vi "Draw.vi"(8 "error in (no error)":errorcluster, 11 "Rectangle in":refnum<class "Rectangle.lvclass">) -> (0 "error out":errorcluster, 2 "Picture":picture, 3 "Rectangle out":refnum<class "Rectangle.lvclass">)   [LabVIEW 2015, in "LV Image Editor Framework.lvlib" / "Rectangle.lvclass"]
uses:
  Rectangle.lvclass
  Shape/Shape.lvclass/Shape.ctl
  Rectangle.lvclass/Rectangle.ctl
  Layered Shape/Layered Shape.lvclass
  Shape/Shape.lvclass
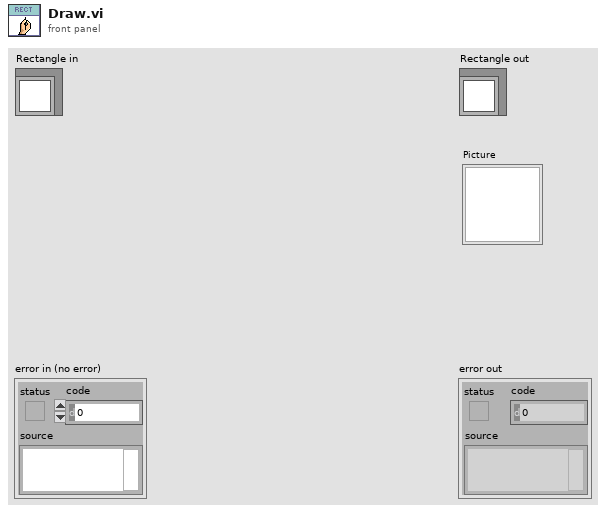
[diagram p1: front panel]
types:
  T1 = cluster{"Left":i32, "Top":i32, "Right":i32, "Bottom":i32}
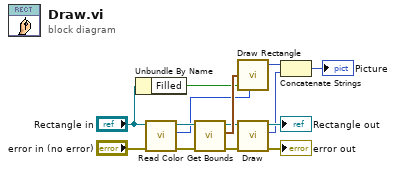
[diagram p0: block diagram]
diagram:
  n1 = Unbundle By Name("Rectangle in") -> ("Filled"=w11:bool)
  n2 = call "Read Color.vi"("error in (no error)"="error in (no error)", "Shape in"="Rectangle in") -> ("error out"=w10:errorcluster, "Color"=w12:u32, "Shape out"=w14:refnum<class "Rectangle.lvclass">)  [unwired: 7 in]
  n3 = call "Get Bounds.vi"("error in (no error)"=w10, "Shape in"=w14) -> ("error out"=w2:errorcluster, "Bounds"=w13:T1, "Shape out"=w7:refnum<class "Rectangle.lvclass">)  [unwired: 7 in]
  n4 = call <vilib>:"Draw Rectangle.vi"("rect"=w13, "fill?(F)"=w11, "color(black)"=w12) -> ("new picture"=w5:picture)  [unwired: 6 in]
  n5 = call-parent "Draw.vi"("error in (no error)"=w2, "Layered Shape in"=w7) -> ("error out"=→"error out":errorcluster, "Picture"=w4:picture, "Layered Shape out"=→"Rectangle out":refnum<class "Rectangle.lvclass">)  [unwired: 7 in]
  n6 = Concatenate Strings(w5, w4) -> (→"Picture":picture)
